vi "getPositionABS.vi"(3 "Device":refnum<k24>) -> (0 "GetPOS":dbl, 1 "Device out":refnum<k24>)   [LabVIEW 2014]
doc: "Returns the <B>absolute position value</B> of motor.\n\n\nAndré Romero - 2017\nandretec@ifsc.usp.br"
uses:
  C:/user-Lab/AndreTec/GITs/andretec/Thorlabs-Vector-Move/kinesisTec/Kinesis/Thorlabs.MotionControl.TCube.DCServoCLI.dll
  kinesisTec/Kinesis/Thorlabs.MotionControl.TCube.DCServoCLI.dll
panel:
  out "GetPositionCounter":i32
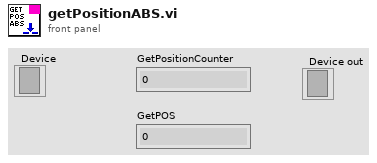
[diagram p1: front panel]
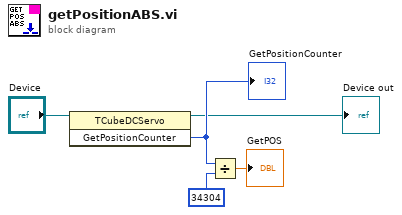
[diagram p0: block diagram]
diagram:
  n1 = invoke class="TCubeDCServo" method="GetPositionCounter"(reference="Device") -> (reference out=→"Device out":refnum<k24>, "GetPositionCounter"=w2:i32)  [unwired: 2 in, 1 out]
  "GetPositionCounter" <- w2
  n2 = Divide(x=w2, y=34304) -> (x/y=→"GetPOS":dbl)
